vi "GamePlayfield_PlaceTetromino.vi"(1 "Origin":i16, 4 "Tetromino":u8, 9 "Player":u8) -> ()   [LabVIEW 2018]
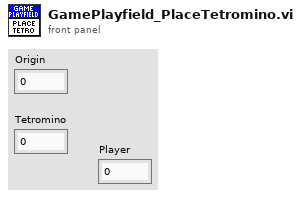
[diagram p1: front panel]
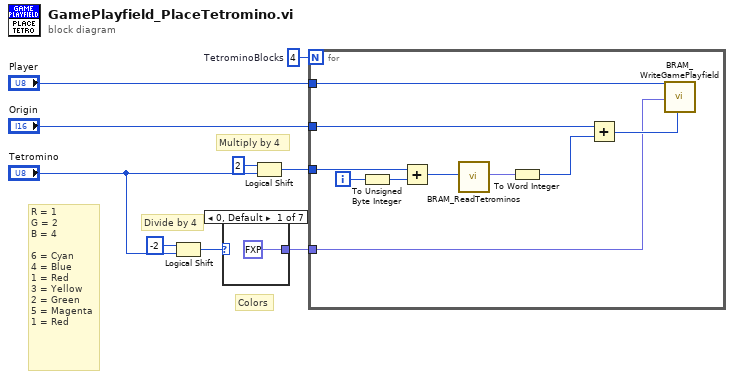
[diagram p0: block diagram]
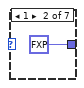
[diagram p2: hidden frame]
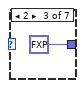
[diagram p3: hidden frame]
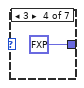
[diagram p4: hidden frame]
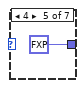
[diagram p5: hidden frame]
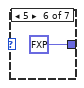
[diagram p6: hidden frame]
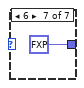
[diagram p7: hidden frame]
diagram:
  w8 = 4  # TetrominoBlocks
  # "Colors"
  # "Divide by 4"
  # "R = 1\nG = 2\nB = 4\n\n6 = Cyan\n4 = Blue\n1 = Red\n3 = Yellow\n2 = Green\n5 = Magenta\n1 = Red"
  # "Multiply by 4"
  n1 = Logical Shift(y=i16 -2, x="Tetromino") -> (x << y=w3:u8)
  n2 = case shown="0, Default" w3 {
    tunnel: [fxp<+,3,3> 6.0 fxp<+,3,3> 4.0 fxp<+,1,1> 1.0 fxp<+,2,2> 3.0 fxp<+,3,3> 2.0 fxp<+,3,3> 5.0 fxp<+,1,1> 1.0] -> w2
    frame 0, Default {
    }
    frame 1 {
    }
    frame 2 {
    }
    frame 3 {
    }
    frame 4 {
    }
    frame 5 {
    }
    frame 6 {
    }
  }
  n3 = Logical Shift(y=i16 2, x="Tetromino") -> (x << y=w7:u8)
  n4 = for {
    N: w8 -> [_]
    tunnel: w7 -> [w26]
    tunnel: "Origin" -> [w23]
    tunnel: w2 -> [w18]
    tunnel: "Player" -> [w17]
    i -> [w25]
    n5 = To Unsigned Byte Integer(number=w25) -> (unsigned 8bit integer=w24:u8)
    n6 = Add(x=w26, y=w24) -> (x+y=w20:u8)
    n7 = call "BRAM_ReadTetrominos.vi"("Address"=w20) -> ("Data"=w22:fxp<+,6,6>)  [unwired: 18 in]
    n8 = To Word Integer(number=w22) -> (16bit integer=w21:i16)
    n9 = Add(x=w23, y=w21) -> (x+y=w19:i16)
    n10 = call "BRAM_WriteGamePlayfield.vi"("Player IN"=w17, "Data"=w18, "Address"=w19) -> ()  [unwired: 16 in, 1 out]
  }
